vi "hmi_status.vi"(7 "hmi_references":T2, 8 "error in (no error)":errorcluster, 10 "action":T1, 11 "build_spec.build_spec_name":string) -> (0 "error out":errorcluster)   [LabVIEW 2015, in "lv-build-interface.lvlib"]
uses:
  lv-build-interface.lvlib
  _controls/hmi_references.ctl
  _controls/action.ctl
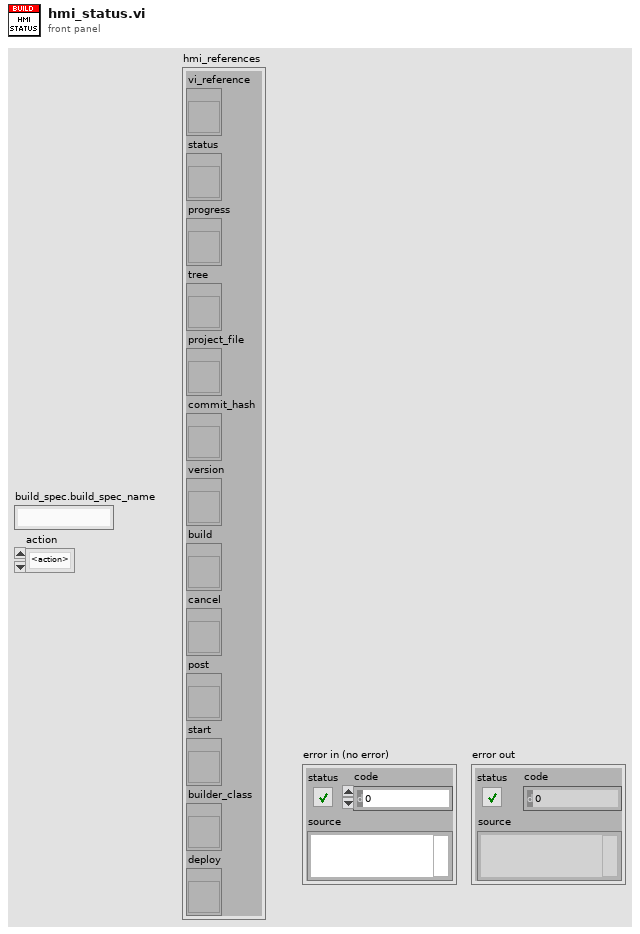
[diagram p1: front panel]
types:
  T1 = typedef "lv-build-interface.lvlib/action.ctl" = enum16{"<action>", "version", "build", "post", "deploy", "<null>"}
  T2 = typedef "lv-build-interface.lvlib/hmi_references.ctl" = cluster{"vi_reference":refnum<vi>, "status":refnum<vi>, "progress":refnum<vi>, "tree":refnum<vi>, "project_file":refnum<vi>, "commit_hash":refnum<vi>, "version":refnum<vi>, "build":refnum<vi>, "cancel":refnum<vi>, "post":refnum<vi>, "start":refnum<vi>, "builder_class":refnum<vi>, "deploy":refnum<vi>}
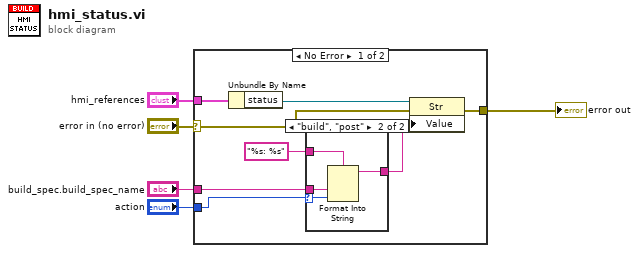
[diagram p0: block diagram]
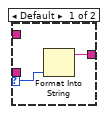
[diagram p2: hidden frame]
diagram:
  n1 = case shown="No Error" "error in (no error)" {
    selector: "error in (no error)" -> [w10 w20]
    tunnel: "hmi_references" -> [w13 _]
    tunnel: [w9 w20] -> w3
    tunnel: "build_spec.build_spec_name" -> [w8 _]
    tunnel: "action" -> [w7 _]
    frame No Error {
      n2 = Unbundle By Name(w13) -> ("status"=w12:refnum<vi>)
      n3 = case shown="\"build\", \"post\"" w7 {
        selector: w7 -> [w15 w18]
        tunnel: w8 -> [_ w19]
        tunnel: [w14 w17] -> w11
        tunnel: "%s: %s" ("format string") -> [_ w16]
        frame Default {
          n4 = Format Into String(w15) -> (resulting string=w14:string)  [unwired: 3 in, 1 out]
        }
        frame "build", "post" {
          n5 = Format Into String(format string=w16, w19, w18) -> (resulting string=w17:string)  [unwired: 2 in, 1 out]
        }
      }
      n6 = property class="Str"(reference=w12, error in=w10, "Value"=w11) -> (error out=w9:errorcluster)  [unwired: 1 out]
    }
    frame Error {
    }
  }
  "error out" <- w3
